vi "Interpolate_1D_Array.vi"(9 "Density Factor":dbl=3.0 format="%#_13g", 11 "x-Axis in":dbl[](array[numeric])) -> (3 "Interpolated Array":dbl[](array[numeric]))   [LabVIEW 2018]
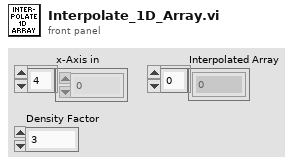
[diagram p1: front panel]
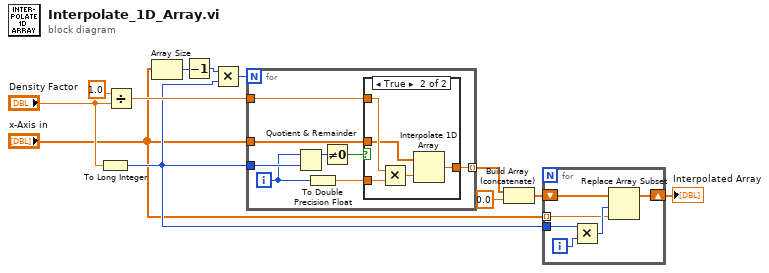
[diagram p0: block diagram]
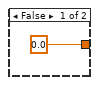
[diagram p2: hidden frame]
diagram:
  n1 = To Long Integer(number="Density Factor") -> (32bit integer=w6:i32)
  n2 = Divide(x=1.0, y="Density Factor") -> (x/y=w11:dbl)
  n3 = Array Size(array="x-Axis in") -> (size(s)=w9:i32)
  n4 = Decrement(x=w9) -> (x-1=w8:i32)
  n5 = Multiply(x=w8, y=w6) -> (x*y=w7:i32)
  n6 = for {
    N: w7 -> [_]
    tunnel: w11 -> [w18]
    tunnel: w6 -> [w20]
    tunnel: "x-Axis in" -> [w14]
    tunnel: [w13] -> w3 mode=indexing
    i -> [w16]
    n7 = Quotient & Remainder(x=w16, y=w20) -> (x-y*floor(x/y)=w19:i32)  [unwired: 1 out]
    n8 = To Double Precision Float(number=w16) -> (double precision float=w15:dbl)
    n9 = Not Equal To 0?(x=w19) -> (x != 0?=w17:bool)
    n10 = case shown="True" w17 {
      tunnel: w14 -> [_ w23]
      tunnel: w18 -> [_ w25]
      tunnel: w15 -> [_ w26]
      tunnel: [0.0 w22] -> w13
      frame False {
      }
      frame True {
        n11 = Multiply(x=w25, y=w26) -> (x*y=w24:dbl)
        n12 = Interpolate 1D Array(1:w24, 2:w23) -> (0:w22:dbl)
      }
    }
  }
  n13 = Build Array (concatenate)(w3, 0.0) -> (w1:dbl[])
  n14 = for {
    tunnel: w6 -> [w31]
    tunnel: "x-Axis in" -> [w28] mode=indexing
    shift-right: [w27] -> w4
    shift-left: w1 -> [w32]
    i -> [w30]
    n15 = Multiply(x=w31, y=w30) -> (x*y=w29:i32)
    n16 = Replace Array Subset(array=w32, new element=w28, index=w29) -> (w27:dbl[])
  }
  "Interpolated Array" <- w4
